vi "move item between listboxes.vi"(8 "error in":errorcluster, 10 "target":refnum<vi>, 11 "source":refnum<vi>) -> (0 "error out":errorcluster, 2 "new target":string[](array[string]), 3 "new source":string[](array[string]))   [LabVIEW 2013, in "TagBusProcessingPluginFeatureDecider.lvclass"]
uses:
  TagBusProcessingPluginFeatureDecider.lvclass
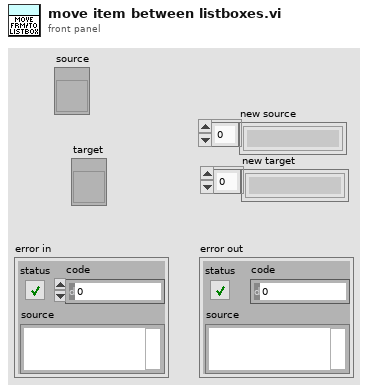
[diagram p1: front panel]
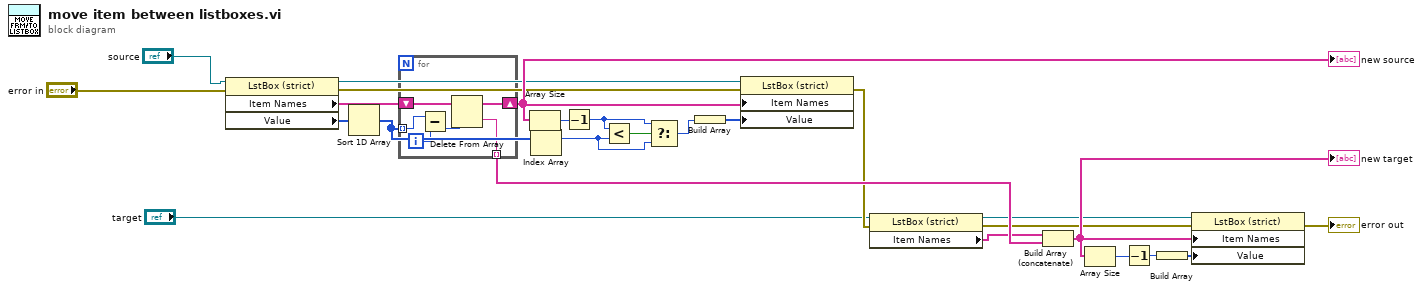
[diagram p0: block diagram]
diagram:
  n1 = property class="LstBox (strict)"(reference="source", error in="error in") -> (reference out=w9:refnum<vi>, error out=w8:errorcluster, "Item Names"=w7:string[], "Value"=w13:i32[])
  n2 = Sort 1D Array(array=w13) -> (sorted array=w3:i32[])
  n3 = for {
    tunnel: [w31] -> w22 mode=indexing
    tunnel: w3 -> [w28] mode=indexing
    shift-right: [w30] -> w10
    shift-left: w7 -> [w29]
    i -> [w26]
    n4 = Subtract(x=w28, y=w26) -> (x-y=w27:i32)
    n5 = Delete From Array(array=w29, index=w27) -> (deleted portion=w31:string, array with subset deleted=w30:string[])  [unwired: 1 in]
  }
  "new source" <- w10
  n6 = Array Size(array=w10) -> (size(s)=w11:i32)
  n7 = Index Array(array=w3) -> (element=w2:i32)  [unwired: 1 in]
  n8 = Decrement(x=w11) -> (x-1=w14:i32)
  n9 = Less?(x=w14, y=w2) -> (x < y?=w12:bool)
  n10 = Select(t=w14, s=w12, f=w2) -> (s? t:f=w15:i32)
  n11 = Build Array(w15) -> (w1:i32[])
  n12 = property class="LstBox (strict)"(reference=w9, error in=w8, "Item Names"=w10, "Value"=w1) -> (error out=w18:errorcluster)  [unwired: 1 out]
  n13 = property class="LstBox (strict)"(reference="target", error in=w18) -> (reference out=w16:refnum<vi>, error out=w17:errorcluster, "Item Names"=w21:string[])
  n14 = Build Array (concatenate)(w21, w22) -> (w23:string[])
  "new target" <- w23
  n15 = Array Size(array=w23) -> (size(s)=w25:i32)
  n16 = Decrement(x=w25) -> (x-1=w24:i32)
  n17 = Build Array(w24) -> (w4:i32[])
  n18 = property class="LstBox (strict)"(reference=w16, error in=w17, "Item Names"=w23, "Value"=w4) -> (error out=→"error out":errorcluster)  [unwired: 1 out]
